vi "HandeFitParams.vi"(6 "Par names":string[](array[string]), 7 "task":T3(ring)=enum."Reset", 8 "error in (no error)":errorcluster, 9 "Pars in":T2(array[cluster]), 10 "Vars in":dbl[](array[numeric]), 11 "tracename in":string="E:\\current VIs\\Vi\\Data\\data_074.tdms: 20") -> (0 "error out":errorcluster, 1 "Pars out":T1(array[cluster]), 2 "Vars out":dbl[](array[numeric]), 3 "tracename out":string="E:\\current VIs\\Vi\\Data\\data_074.tdms: 20")   [LabVIEW 2018]
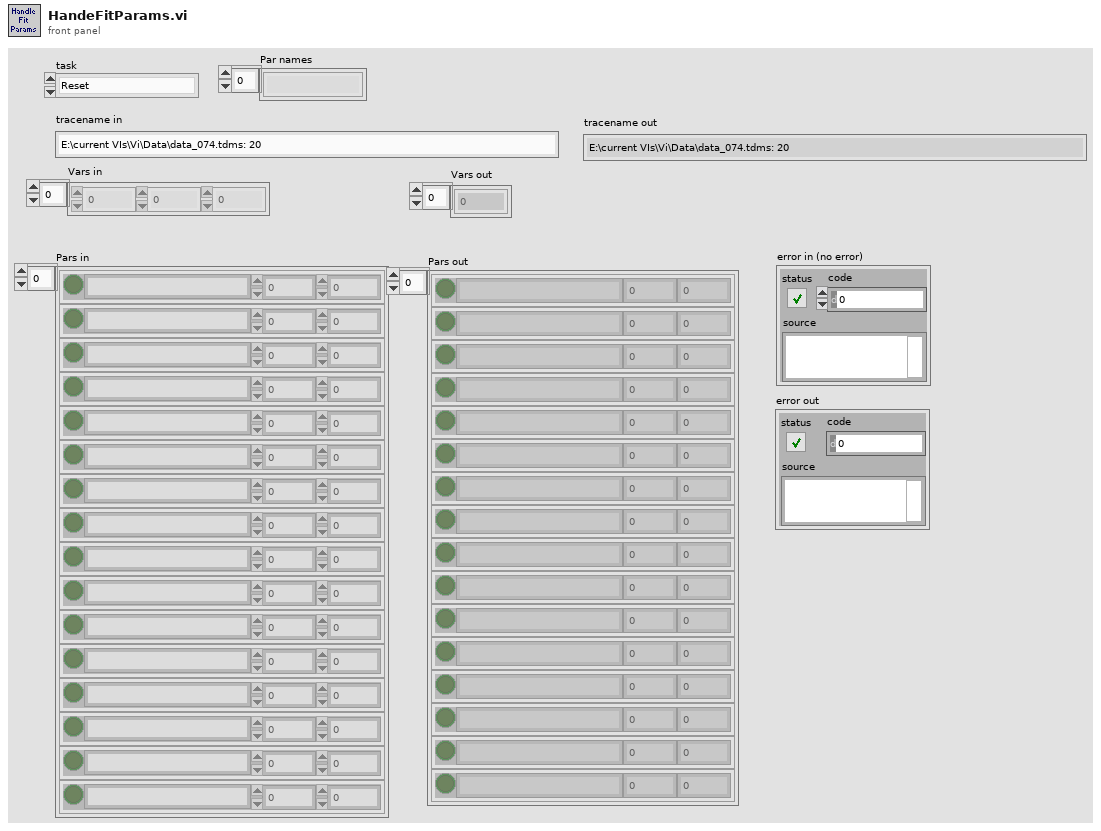
[diagram p1: front panel]
types:
  T1 = cluster{bool, "ParName":string, "Value":dbl, "SE":dbl}[]
  T2 = cluster{"Fit?":bool, "ParName":string, "Value":dbl, "SE":dbl}[]
  T3 = enum16{"Init", "Reset", "Update var pars", "Update SE's", "Get", "Save to file", "Read from file"}
  T4 = cluster{bool, string, "Numeric":dbl, "Numeric":dbl}
  T5 = cluster{"Fit?":bool, "ParName":string, "Value":dbl, "SE":dbl}
  T6 = cluster{bool, "ParName":string, "Value":dbl, "Value":dbl}
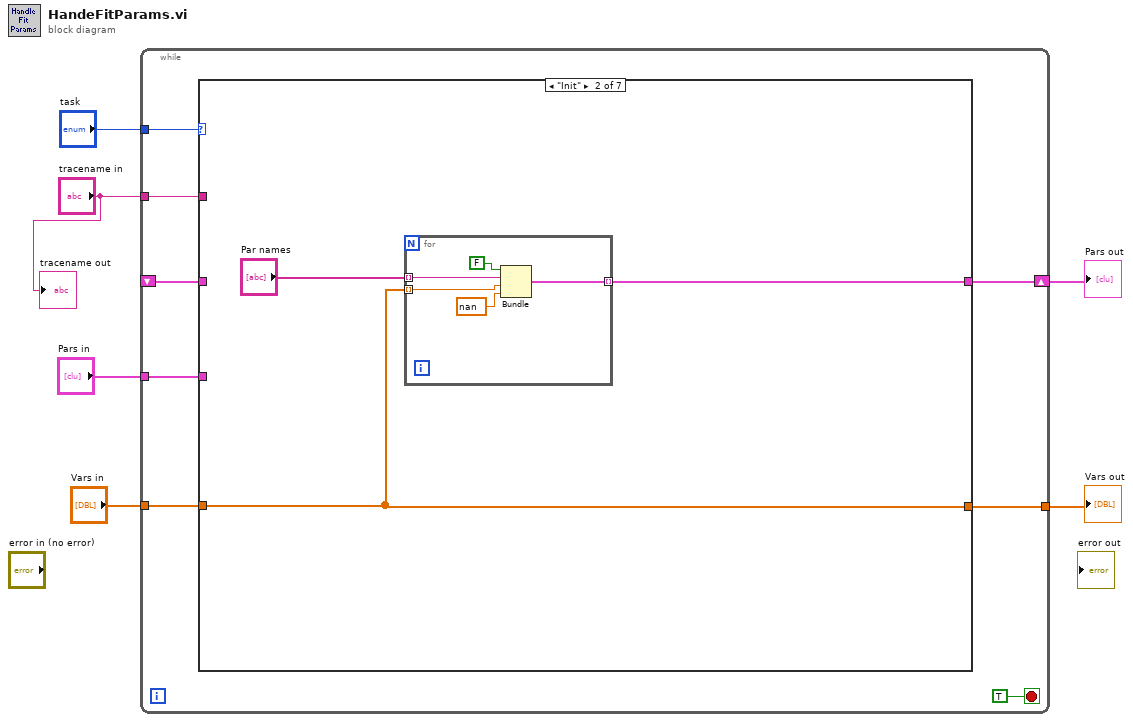
[diagram p0: block diagram]
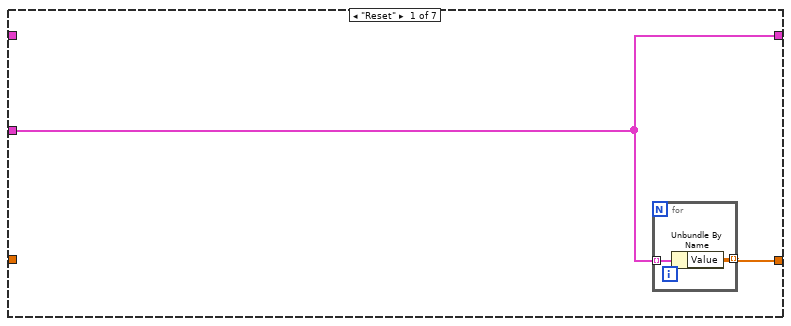
[diagram p2: hidden frame]
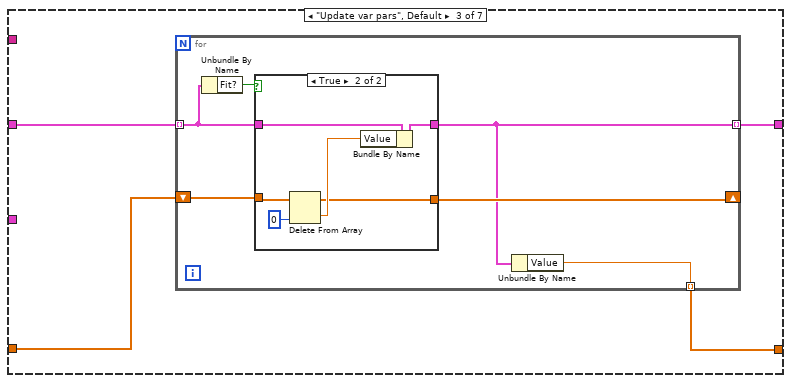
[diagram p3: hidden frame]
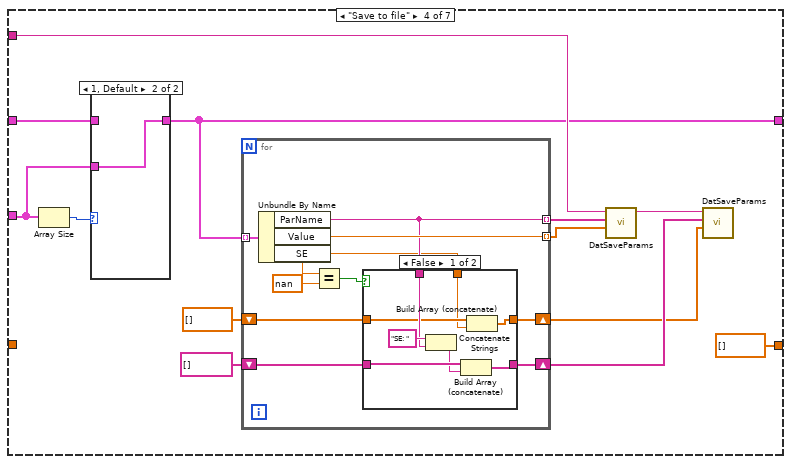
[diagram p5: hidden frame]
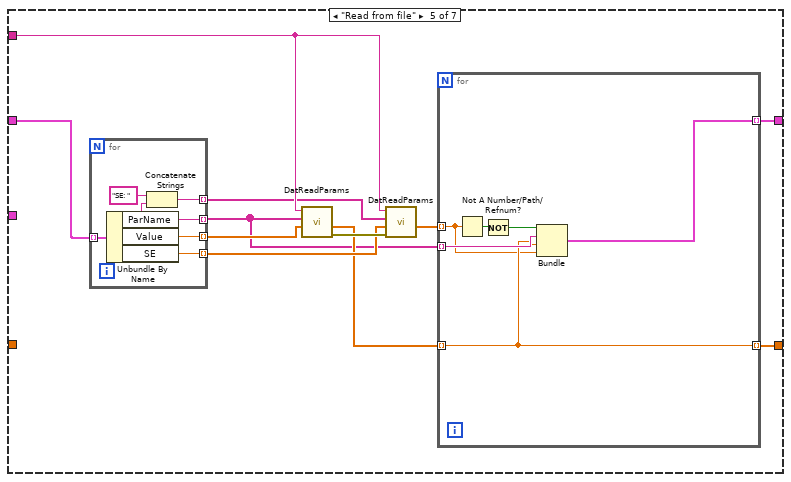
[diagram p8: hidden frame]
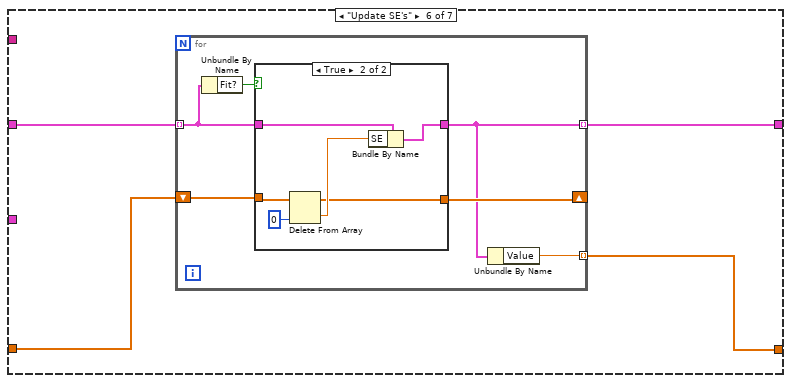
[diagram p9: hidden frame]
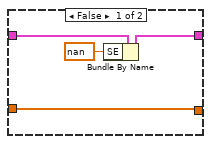
[diagram p10: hidden frame]
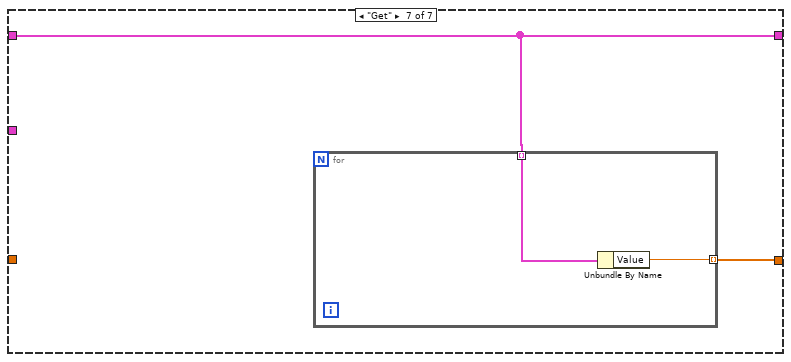
[diagram p11: hidden frame]
diagram:
  n1 = while {
    tunnel: "task" -> [w14]
    shift-right: [w12] -> w5
    shift-left: _ -> [w10]
    tunnel: "Vars in" -> [w11]
    tunnel: [w9] -> w3
    tunnel: "tracename in" -> [w8]
    tunnel: "Pars in" -> [w7]
    stop <- TRUE stop-if-true
    n2 = case shown="\"Init\"" w14 {
      tunnel: [w15 w20 w29 w47 w80 w105 w124] -> w12
      tunnel: [w16 w21 w28 dbl[] [] w84 w104 w123] -> w9
      tunnel: w11 -> [_ w21 w30 _ _ w106 _]
      tunnel: w10 -> [_ _ w27 w46 w81 w103 w124]
      tunnel: w8 -> [_ _ _ w54 w89 _ _]
      tunnel: w7 -> [w15 _ _ w45 _ _ _]
      frame "Reset" {
        n3 = for {
          tunnel: w15 -> [w18] mode=indexing
          tunnel: [w17] -> w16 mode=indexing
          n4 = Unbundle By Name(w18) -> ("Value"=w17:dbl)
        }
      }
      frame "Init" {
        n5 = for {
          tunnel: w21 -> [w26] mode=indexing
          tunnel: "Par names" -> [w25] mode=indexing
          tunnel: [w22] -> w20 mode=indexing
          n6 = Bundle(FALSE, w25, "Numeric"=w26, "Numeric"=nan) -> (w22:T4)  [unwired: 1 in]
        }
      }
      frame "Update var pars", Default {
        n7 = for {
          shift-right: [w33] -> _
          shift-left: w30 -> [w34]
          tunnel: w27 -> [w35] mode=indexing
          tunnel: [w32] -> w29 mode=indexing
          tunnel: [w31] -> w28 mode=indexing
          n8 = Unbundle By Name(w35) -> ("Fit?"=w36:bool)
          n9 = case shown="True" w36 {
            tunnel: w35 -> [w38 w44]
            tunnel: w34 -> [w37 w43]
            tunnel: [w37 w40] -> w33
            tunnel: [w38 w39] -> w32
            frame False {
            }
            frame True {
              n10 = Delete From Array(array=w43, index=0) -> (deleted portion=w41:dbl, array with subset deleted=w40:dbl[])  [unwired: 1 in]
              n11 = Bundle By Name(cluster=w44, "Value"=w41) -> (w39:T5)
            }
          }
          n12 = Unbundle By Name(w32) -> ("Value"=w31:dbl)
        }
      }
      frame "Save to file" {
        n13 = Array Size(array=w45) -> (size(s)=w48:i32)
        n14 = case shown="1, Default" w48 {
          tunnel: [w58 w59] -> w47
          tunnel: w46 -> [w58 _]
          tunnel: w45 -> [_ w59]
          frame 0 {
          }
          frame 1, Default {
          }
        }
        n15 = for {
          tunnel: w47 -> [w62] mode=indexing
          tunnel: [w61] -> w53 mode=indexing
          tunnel: [w69] -> w52 mode=indexing
          shift-right: [w66] -> w49
          shift-left: dbl[] [] -> [w65]
          shift-right: [w64] -> w50
          shift-left: string[] [] -> [w63]
          n16 = Unbundle By Name(w62) -> ("ParName"=w61:string, "Value"=w69:dbl, "SE"=w60:dbl)
          n17 = Equal?(x=w60, y=nan) -> (x = y?=w67:bool)
          n18 = case shown="False" w67 {
            tunnel: [w70 w79] -> w66
            tunnel: w65 -> [w72 w79]
            tunnel: [w75 w78] -> w64
            tunnel: w63 -> [w76 w78]
            tunnel: w61 -> [w74 _]
            tunnel: w60 -> [w71 _]
            frame False {
              n19 = Concatenate Strings("SE: " ("string"), w74) -> (w73:string)
              n20 = Build Array (concatenate)(w76, w73) -> (w75:string[])
              n21 = Build Array (concatenate)(w72, w71) -> (w70:dbl[])
            }
            frame True {
            }
          }
        }
        n22 = call "DatSaveParams.vi"("Values"=w52, "Names"=w53, "tracename"=w54) -> ("tracename out"=w51:string)  [unwired: 5 in, 1 out]
        n23 = call "DatSaveParams.vi"("Values"=w49, "Names"=w50, "tracename"=w51) -> ()  [unwired: 5 in, 2 out]
      }
      frame "Read from file" {
        n24 = for {
          tunnel: w81 -> [w102] mode=indexing
          tunnel: [w100] -> w82 mode=indexing
          tunnel: [w99] -> w83 mode=indexing
          tunnel: [w98] -> w88 mode=indexing
          tunnel: [w97] -> w87 mode=indexing
          n25 = Unbundle By Name(w102) -> ("ParName"=w100:string, "Value"=w99:dbl, "SE"=w97:dbl)
          n26 = Concatenate Strings("SE: " ("string"), w100) -> (w98:string)
        }
        n27 = call "DatReadParams.vi"("default Values"=w83, "Names"=w82, "tracename"=w89) -> ("error out"=w90:errorcluster, "Values out"=w85:dbl[])  [unwired: 4 in, 1 out]
        n28 = call "DatReadParams.vi"("error in (no error)"=w90, "default Values"=w87, "Names"=w88, "tracename"=w89) -> ("Values out"=w86:dbl[])  [unwired: 3 in, 2 out]
        n29 = for {
          tunnel: w86 -> [w92] mode=indexing
          tunnel: w85 -> [w93] mode=indexing
          tunnel: [w93] -> w84 mode=indexing
          tunnel: w82 -> [w94] mode=indexing
          tunnel: [w91] -> w80 mode=indexing
          n30 = Not A Number/Path/Refnum?(number/path/refnum=w92) -> (NaN/Path/Refnum?=w96:bool)
          n31 = Not(x=w96) -> (.not. x?=w95:bool)
          n32 = Bundle(w95, "ParName"=w94, "Value"=w93, "Value"=w92) -> (w91:T6)  [unwired: 1 in]
        }
      }
      frame "Update SE's" {
        n33 = for {
          shift-right: [w109] -> _
          shift-left: w106 -> [w110]
          tunnel: w103 -> [w111] mode=indexing
          tunnel: [w108] -> w105 mode=indexing
          tunnel: [w107] -> w104 mode=indexing
          n34 = Unbundle By Name(w111) -> ("Fit?"=w112:bool)
          n35 = case shown="True" w112 {
            tunnel: w111 -> [w116 w122]
            tunnel: w110 -> [w115 w121]
            tunnel: [w115 w118] -> w109
            tunnel: [w114 w117] -> w108
            frame False {
              n36 = Bundle By Name(cluster=w116, "SE"=nan) -> (w114:T5)
            }
            frame True {
              n37 = Delete From Array(array=w121, index=0) -> (deleted portion=w119:dbl, array with subset deleted=w118:dbl[])  [unwired: 1 in]
              n38 = Bundle By Name(cluster=w122, "SE"=w119) -> (w117:T5)
            }
          }
          n39 = Unbundle By Name(w108) -> ("Value"=w107:dbl)
        }
      }
      frame "Get" {
        n40 = for {
          tunnel: w124 -> [w126] mode=indexing
          tunnel: [w125] -> w123 mode=indexing
          n41 = Unbundle By Name(w126) -> ("Value"=w125:dbl)
        }
      }
    }
  }
  "Vars out" <- w3
  "Pars out" <- w5
  "tracename out" <- "tracename in"
